vi "Create Clip Plane.vi"(8 "error in (no error)":errorcluster, 10 "Number":i32, 11 "Plane":cluster{"A":sgl, "B":sgl, "C":sgl, "D":sgl}) -> (0 "error out":errorcluster, 3 "New Clip Plane Refnum":refnum<vi>)   [LabVIEW 2020, in "NI_3D Picture Control.lvlib"]
doc: "Defines a plane in the 3D scene beyond which objects cannot be drawn."
uses:
  <vilib>/picture/3D Picture Control/NI_3D Picture Control.lvlib
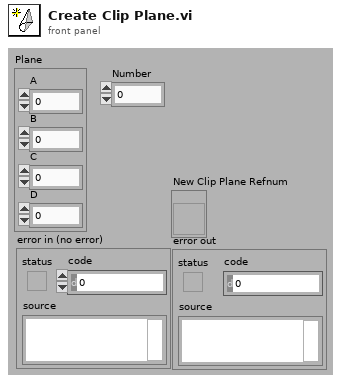
[diagram p1: front panel]
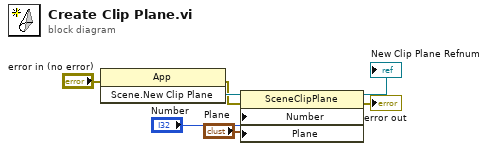
[diagram p0: block diagram]
diagram:
  n1 = invoke class="App" method="Scene.New Clip Plane"(error in="error in (no error)") -> (error out=w6:errorcluster, "Scene.New Clip Plane"=w7:refnum<vi>)  [unwired: 2 in, 1 out]
  n2 = property class="SceneClipPlane"(reference=w7, error in=w6, "Number"="Number", "Plane"="Plane") -> (reference out=→"New Clip Plane Refnum":refnum<vi>, error out=→"error out":errorcluster)
